vi "Result_Test.vi"(8 "error in (no error)":errorcluster caption="entrée d'erreur (pas d'erreur)", 11 "Get_Voltage en entrée":refnum<class "Get_Addr_Mac_DB_AIS.lvclass">) -> (0 "error out":errorcluster caption="sortie d'erreur", 3 "Get_Voltage en sortie":refnum<class "Get_Addr_Mac_DB_AIS.lvclass">)   [LabVIEW 2020, in "Library Test.lvlib" / "Get_Addr_Mac_DB_AIS.lvclass"]
uses:
  Get_Addr_Mac_DB_AIS.lvclass
  C:/Users/ngarcin/OneDrive - Altyor/Standard TB/Class/Test/Test (Default)/Test (Default).lvclass
  Find_SN_In_Database/Find_SN_In_Database.lvclass
  Get_Addr_Mac_DB_AIS.lvclass/Get_Addr_Mac_DB_AIS.ctl
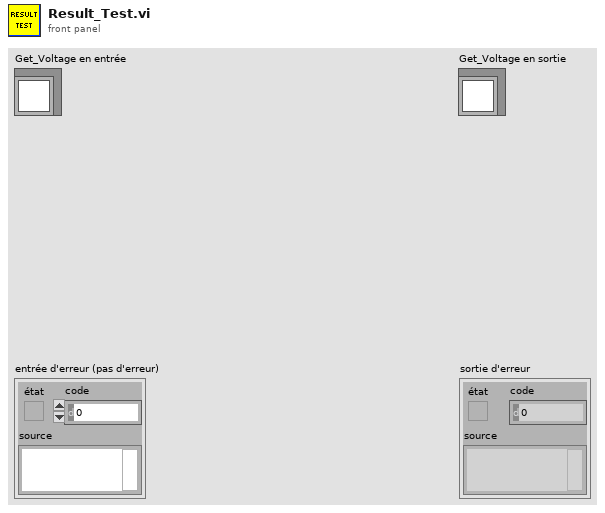
[diagram p1: front panel]
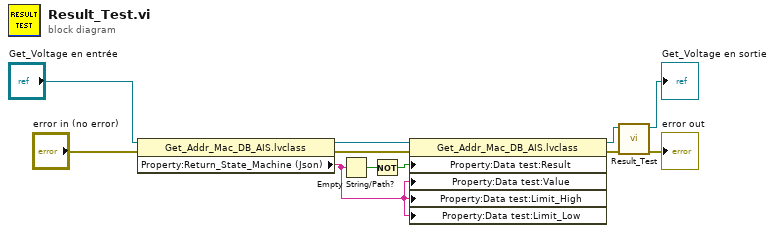
[diagram p0: block diagram]
diagram:
  n1 = property class="Get_Addr_Mac_DB_AIS.lvclass"(reference="Get_Voltage en entrée", error in="error in (no error)") -> (reference out=w9:refnum<class "Get_Addr_Mac_DB_AIS.lvclass">, error out=w7:errorcluster, "Property:Return_State_Machine (Json)"=w8:string)
  n2 = Empty String/Path?(string/path=w8) -> (empty?=w6:bool)
  n3 = Not(x=w6) -> (.not. x?=w5:bool)
  n4 = property class="Get_Addr_Mac_DB_AIS.lvclass"(reference=w9, error in=w7, "Property:Data test:Result"=w5, "Property:Data test:Value"=w8, "Property:Data test:Limit_High"=w8, "Property:Data test:Limit_Low"=w8) -> (reference out=w2:refnum<class "Get_Addr_Mac_DB_AIS.lvclass">, error out=w1:errorcluster)
  n5 = call-parent "Result_Test.vi"("error in (no error)"=w1, "Generate_SN en entrée"=w2) -> ("error out"=→"error out":errorcluster, "Generate_SN en sortie"=→"Get_Voltage en sortie":refnum<class "Get_Addr_Mac_DB_AIS.lvclass">)  [unwired: 8 in]
